vi "Lab4.vi"() -> ()   [LabVIEW 2021]
panel:
  out "Waveform Chart 2":dynamicdata(graph)
  in  "Frequency":dbl(slide) scale=0.0..5.0
  in  "Amplitude":dbl(slide) scale=0.0..10.0
  out "Waveform Chart":dbl(graph)
  in  "stop":bool
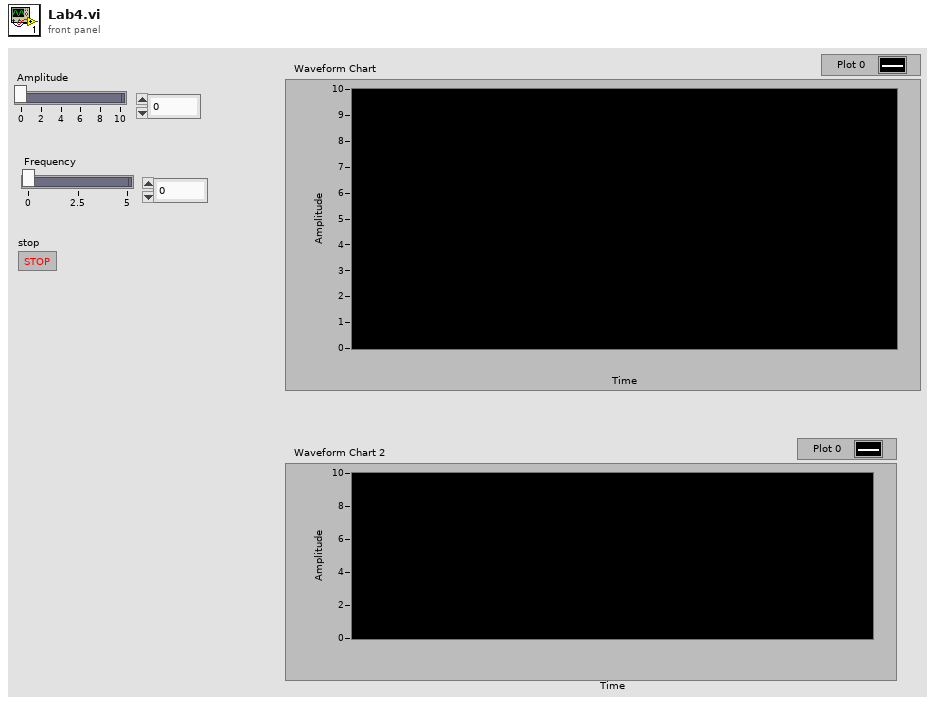
[diagram p1: front panel]
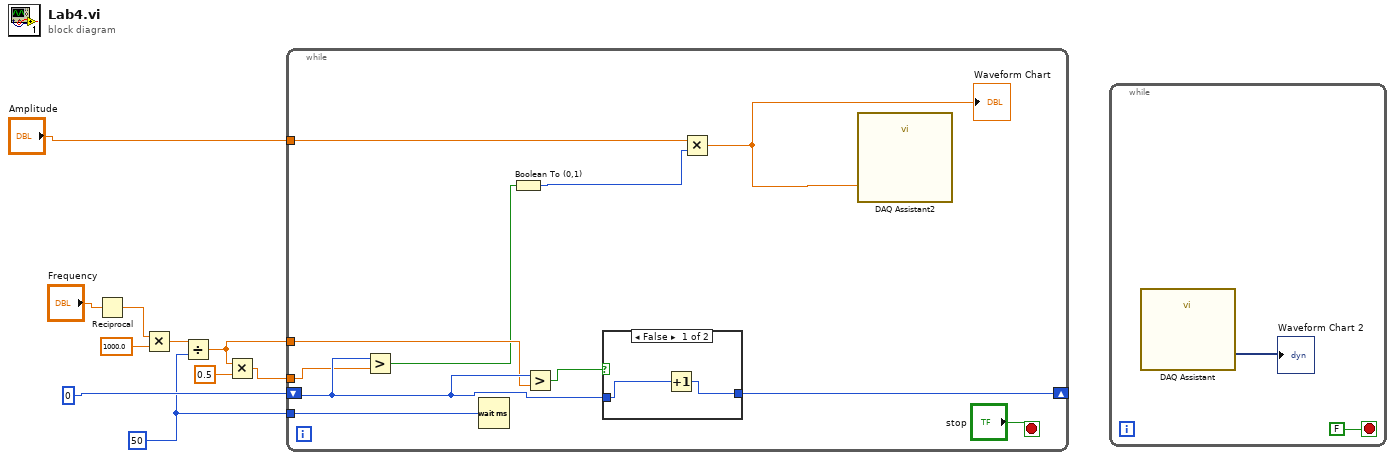
[diagram p0: block diagram]
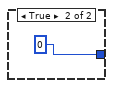
[diagram p2: hidden frame]
diagram:
  w1 = 50
  n1 = Reciprocal(x="Frequency") -> (1/x=w8:dbl)
  n2 = Multiply(x=w8, y=1000.0) -> (x*y=w3:dbl)
  n3 = Divide(x=w3, y=w1) -> (x/y=w2:dbl)
  n4 = Multiply(x=w2, y=0.5) -> (x*y=w4:dbl)
  n5 = while {
    shift-right: [w20] -> _
    shift-left: 0 -> [w18]
    tunnel: "Amplitude" -> [w15]
    tunnel: w2 -> [w14]
    tunnel: w4 -> [w13]
    tunnel: w1 -> [w11]
    stop <- "stop" stop-if-true
    n6 = Greater?(x=w18, y=w13) -> (0:w12:bool)
    n7 = Wait (ms)(milliseconds to wait=w11) -> ()  [unwired: 1 out]
    n8 = Boolean To (0,1)(Boolean=w12) -> (0, 1=w16:i16)
    n9 = Greater?(x=w18, y=w14) -> (0:w21:bool)
    n10 = case shown="False" w21 {
      tunnel: [w23 0] -> w20
      tunnel: w18 -> [w22 _]
      frame False {
        n11 = Increment(x=w22) -> (x+1=w23:i32)
      }
      frame True {
      }
    }
    n12 = Multiply(x=w15, y=w16) -> (x*y=w17:dbl)
    "Waveform Chart" <- w17
    n13 = call "DAQ Assistant2"("data"=w17) -> ()  [unwired: 17 in, 2 out]
  }
  n14 = while {
    stop <- FALSE stop-if-true
    n15 = call "DAQ Assistant"() -> ("data"=→"Waveform Chart 2":dynamicdata)  [unwired: 17 in, 2 out]
  }
